vi "CRYDelete Channel Info.vi"(9 "Channel Info In":T1[](array[typedef]) {"Coupling" items=["Default"=-1, "RSE"=10083, "NRSE"=10078, "Differential"=10106, "Pseudodifferential"=12529]; "term config" items=["Default"=-1, "RSE"=10083, "NRSE"=10078, "Differential"=10106, "Pseudodifferential"=12529]; "Anti-aliasing Factor (%fs)" format="%.2f"}, 11 "Selected Index":u16) -> (1 "Channel Info Out":T1[](array[typedef]) {"Coupling" items=["Default"=-1, "RSE"=10083, "NRSE"=10078, "Differential"=10106, "Pseudodifferential"=12529]; "term config" items=["Default"=-1, "RSE"=10083, "NRSE"=10078, "Differential"=10106, "Pseudodifferential"=12529]; "Anti-aliasing Factor (%fs)" format="%.2f"}, 2 "Name Array":string[](array[string]), 3 "New Index":u16)   [LabVIEW 2013]
uses:
  Typedef Control/CRYHardware Channel Info.ctl
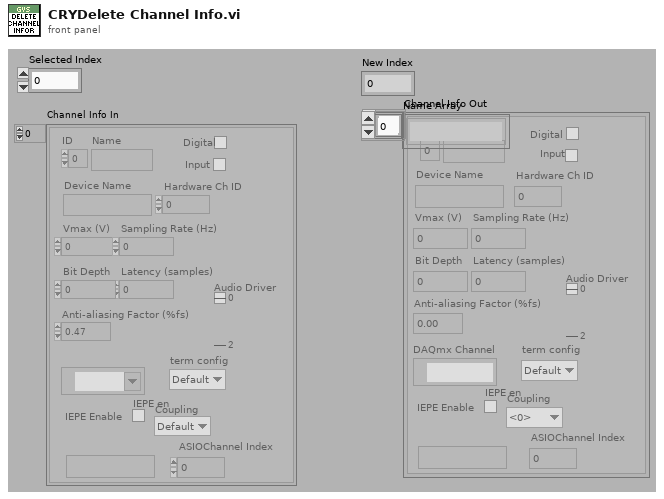
[diagram p1: front panel]
types:
  T1 = typedef "CRYHardware Channel Info.ctl" = cluster{"ID":i32, "Name":string, "Digital":bool, "Input":bool, "Device Name":string, "Hardware Ch ID":u8, "Vmax (V)":dbl, "Latency (samples)":dbl, "Sampling Rate (Hz)":u32, "Bit Depth":u32, "Anti-aliasing Factor (%fs)":sgl, "DAQmx Channel":tag, "term config":i32, "Coupling":i32, "IEPE en":bool, "ASIOChannel Name":string, "Audio Driver":u16, "ASIOChannel Index":u8}
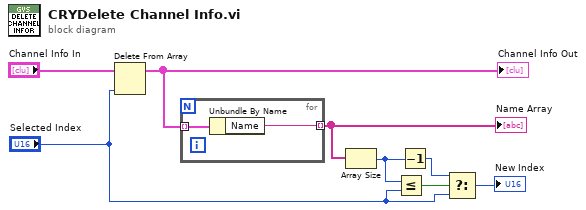
[diagram p0: block diagram]
diagram:
  n1 = Delete From Array(array="Channel Info In", index="Selected Index") -> (array with subset deleted=w8:T1[])  [unwired: 1 in, 1 out]
  "Channel Info Out" <- w8
  n2 = for {
    tunnel: w8 -> [w10] mode=indexing
    tunnel: [w9] -> w4 mode=indexing
    n3 = Unbundle By Name(w10) -> ("Name"=w9:string)
  }
  "Name Array" <- w4
  n4 = Array Size(array=w4) -> (size(s)=w6:i32)
  n5 = Less Or Equal?(x=w6, y="Selected Index") -> (x <= y?=w7:bool)
  n6 = Decrement(x=w6) -> (x-1=w5:i32)
  n7 = Select(t=w5, s=w7, f="Selected Index") -> (s? t:f=→"New Index":i32)
